vi "Compile Static Commands.vi"(10 "State Loop Data in":T1) -> (2 "State Loop Data out":T1)   [LabVIEW 2023, in "VolatusSeq.lvlib" / "State.lvclass"]
uses:
  State.lvclass
  State.lvclass/State.ctl
  Iteration Actions/Iteration Actions.lvclass
  VolatusSeqConfig/Command Type.ctl
  VolatusSeqConfig/VolatusSeqConfig.lvlib
  Volatus/MessageQ/MessageQ.lvclass
  messages/CmdDigital/Data.ctl
  messages/CmdDigital/CmdDigital.lvlib
  messages/CmdAnalog/Data.ctl
  messages/CmdAnalog/CmdAnalog.lvlib
  Command.ctl
  VolatusSeq.lvlib
  Transition/Transition.lvclass
  Sequence Time.ctl
  State Loop Data.ctl
  Send Type.ctl
  Variables/Variables.lvclass
  lv-vecto/Vecto/Channel DBL/Channel DBL.lvclass
  Format String/Format String.lvclass
  VolatusSeqConfig/Debug Flags.ctl
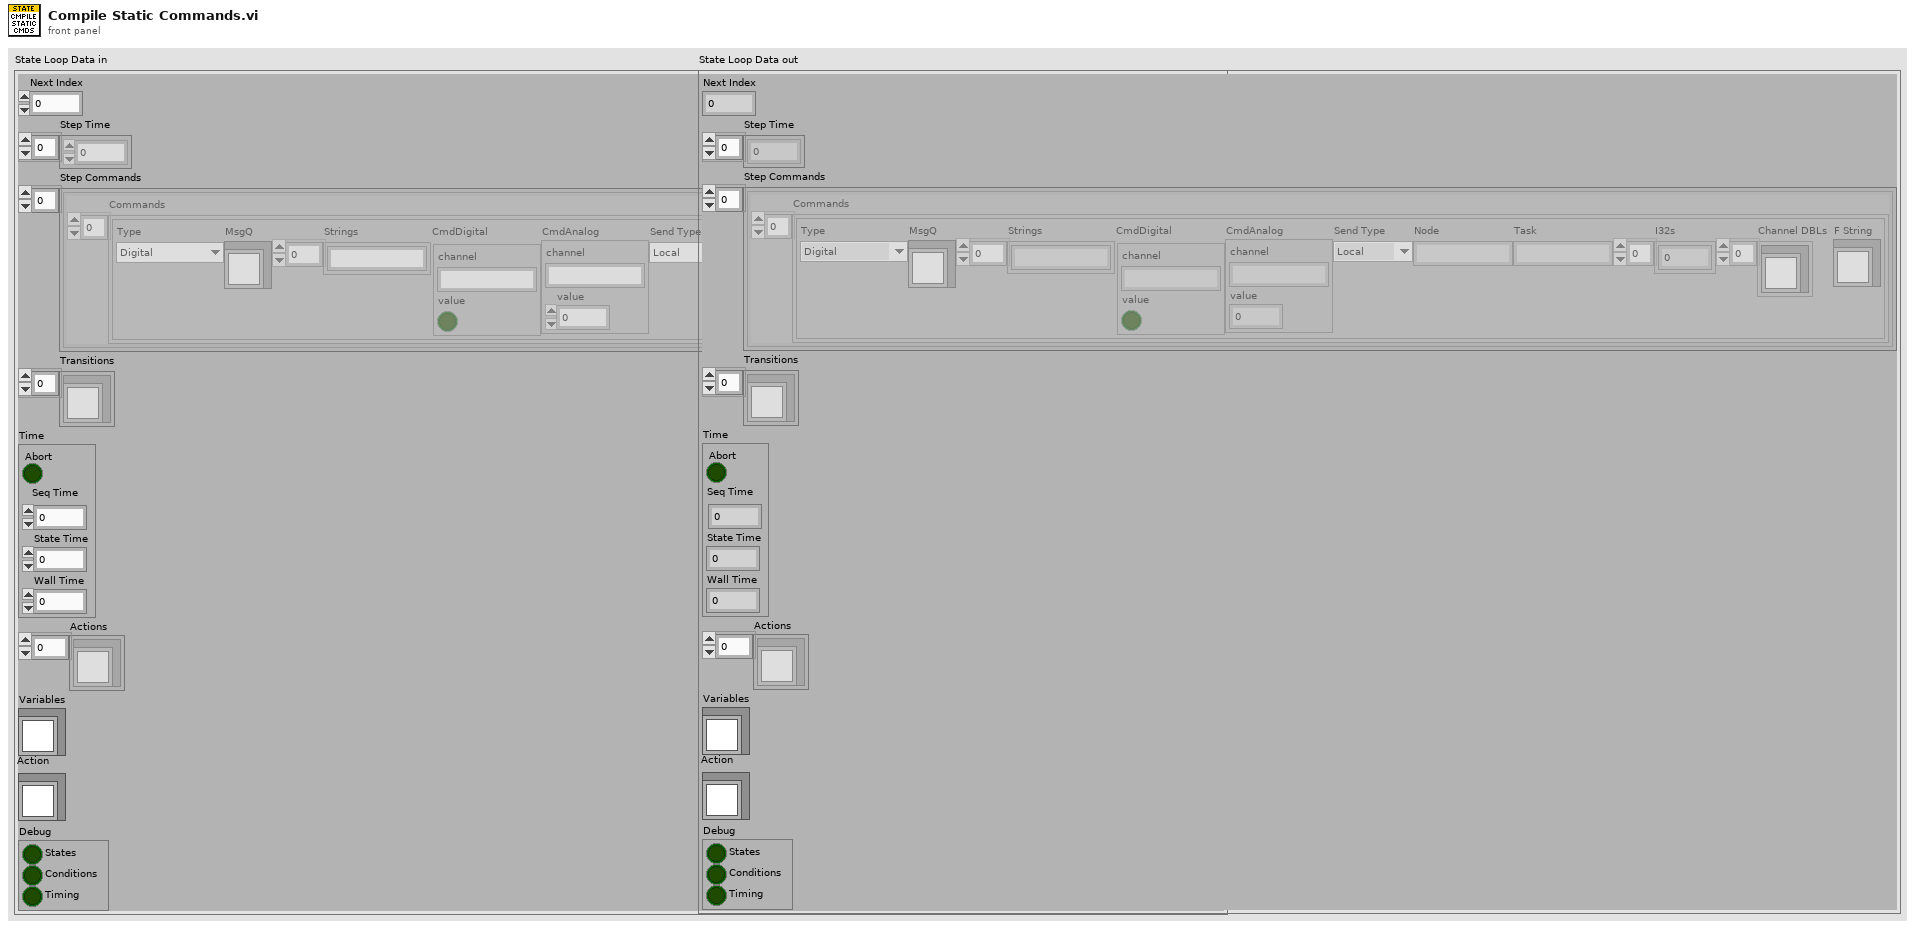
[diagram p1: front panel]
types:
  T1 = typedef "VolatusSeq.lvlib/State.lvclass/State Loop Data.ctl" = cluster{"Next Index":i32, "Step Time":dbl[], "Step Commands":cluster{"Commands":T2[]}[], "Transitions":refnum<class "Transition.lvclass">[], "Time":T7, "Actions":refnum<class "Iteration Actions.lvclass">[], "Variables":refnum<class "Variables.lvclass">, "Action":refnum<class "Iteration Actions.lvclass">, "Debug":T8}
  T2 = typedef "VolatusSeq.lvlib/Command.ctl" = cluster{"Type":T3, "MsgQ":refnum<class "MessageQ.lvclass">, "Strings":string[], "CmdDigital":T4, "CmdAnalog":T5, "Send Type":T6, "Node":string, "Task":string, "I32s":i32[], "Channel DBLs":refnum<class "Channel DBL.lvclass">[], "F String":refnum<class "Format String.lvclass">}
  T3 = typedef "VolatusSeqConfig.lvlib/Command Type.ctl" = enum16{"Digital", "Numeric", "Transition", "Stop", "StartLog", "StopLog", "Start", "Event", "Error", "HTTP", "ResetVar", "IncVar", "DecVar", "SaveVar", "LoadVar", "AddVar", "SubVar", "SetVar", "AddToVar"}
  T4 = typedef "CmdDigital.lvlib/Data.ctl" = cluster{"channel":string, "value":bool}
  T5 = typedef "CmdAnalog.lvlib/Data.ctl" = cluster{"channel":string, "value":dbl}
  T6 = typedef "VolatusSeq.lvlib/Send Type.ctl" = enum16{"Local", "Remote"}
  T7 = typedef "VolatusSeq.lvlib/Sequence Time.ctl" = cluster{"Abort":bool, "Seq Time":dbl, "State Time":dbl, "Wall Time":dbl}
  T8 = typedef "VolatusSeqConfig.lvlib/Debug Flags.ctl" = cluster{"States":bool, "Conditions":bool, "Timing":bool}
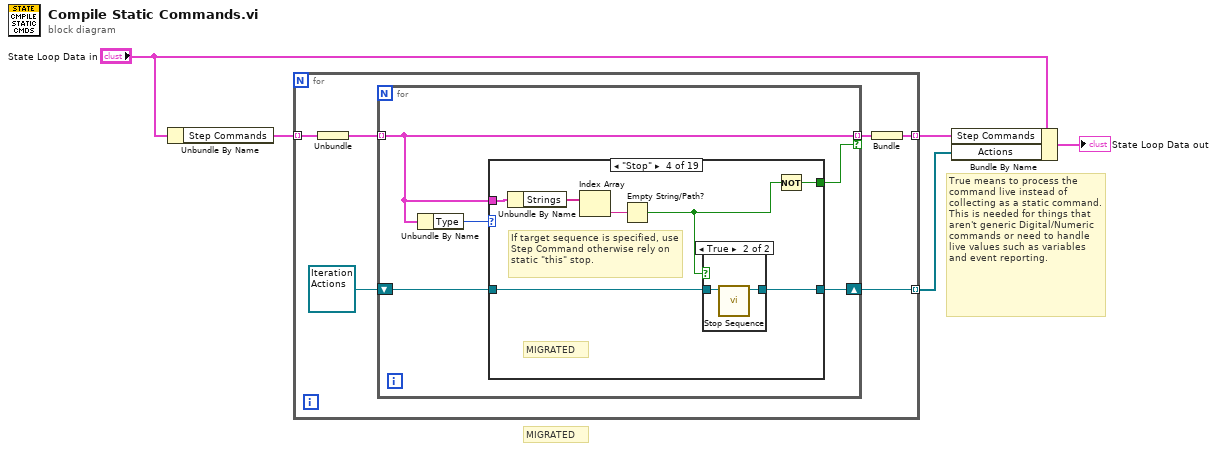
[diagram p0: block diagram]
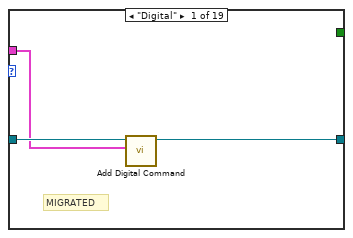
[diagram p2: hidden frame]
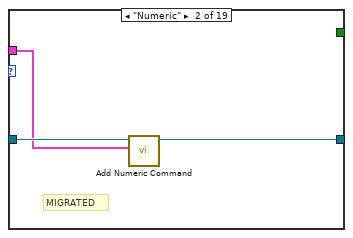
[diagram p3: hidden frame]
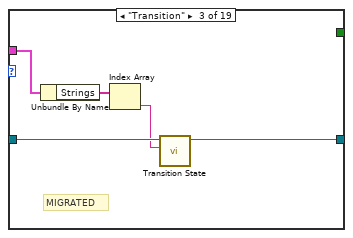
[diagram p4: hidden frame]
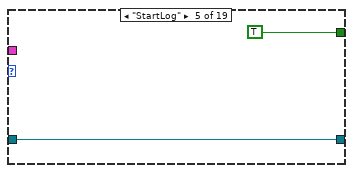
[diagram p6: hidden frame]
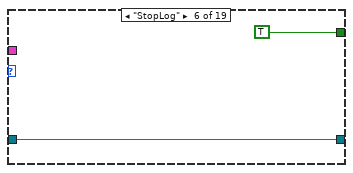
[diagram p7: hidden frame]
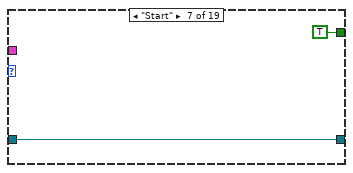
[diagram p8: hidden frame]
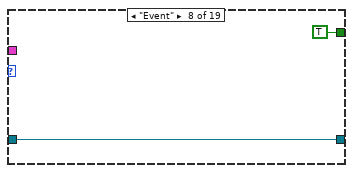
[diagram p9: hidden frame]
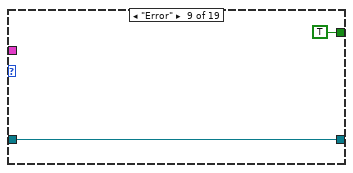
[diagram p10: hidden frame]
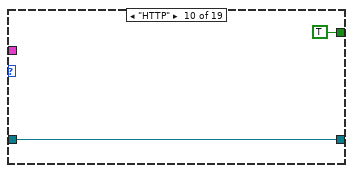
[diagram p11: hidden frame]
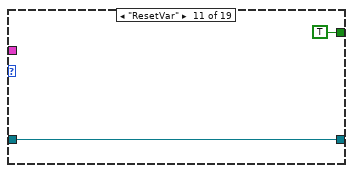
[diagram p12: hidden frame]
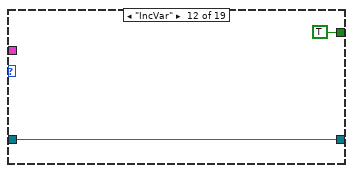
[diagram p13: hidden frame]
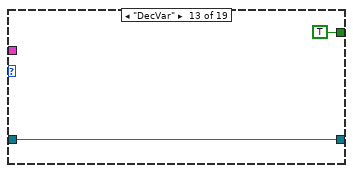
[diagram p14: hidden frame]
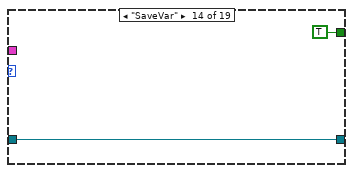
[diagram p15: hidden frame]
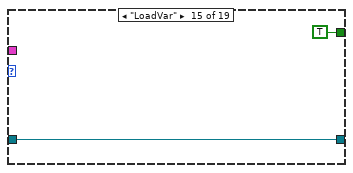
[diagram p16: hidden frame]
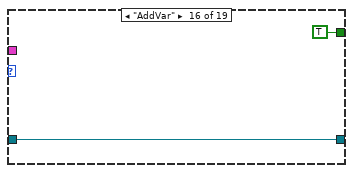
[diagram p17: hidden frame]
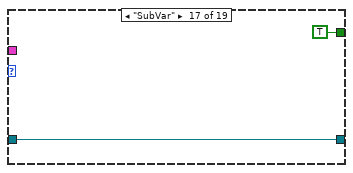
[diagram p18: hidden frame]
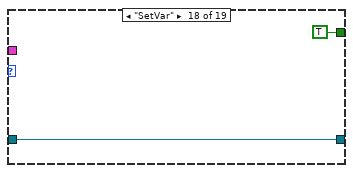
[diagram p19: hidden frame]
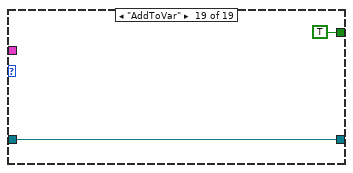
[diagram p20: hidden frame]
diagram:
  # "MIGRATED"
  # "True means to process the command live instead of collecting as a static command. This is needed for things that aren't generic Digital/Numeric commands or need to handle live values such as variables and event reporting."
  n1 = Unbundle By Name("State Loop Data in") -> ("Step Commands"=w3:cluster{"Commands":T2[]}[])
  n2 = for {
    tunnel: w3 -> [w11] mode=indexing
    tunnel: [w7] -> w2 mode=indexing
    tunnel: [w6] -> w1 mode=indexing
    n3 = Unbundle(w11) -> ("Commands"=w10:T2[])
    n4 = for {
      tunnel: w10 -> [w15] mode=indexing
      shift-right: [w13] -> w6
      shift-left: refnum<class "Iteration Actions.lvclass"> refnum ("VolatusSeq.lvlib:Iteration Actions.lvclass") -> [w14]
      tunnel: [w15] -> w8 mode=indexing if=w12
      n5 = Unbundle By Name(w15) -> ("Type"=w16:T3)
      n6 = case shown="\"Stop\"" w16 {
        tunnel: w15 -> [w17 w20 w26 w32 _ _ _ _ _ _ _ _ _ _ _ _ _ _ _]
        tunnel: w14 -> [w19 w22 w27 w34 w39 w41 w43 w45 w47 w49 w51 w53 w55 w57 w59 w61 w63 w65 w67]
        tunnel: [w18 w21 w23 w33 w39 w41 w43 w45 w47 w49 w51 w53 w55 w57 w59 w61 w63 w65 w67] -> w13
        tunnel: [_ _ _ w29 TRUE TRUE TRUE TRUE TRUE TRUE TRUE TRUE TRUE TRUE TRUE TRUE TRUE TRUE TRUE] -> w12
        frame "Digital" {
          # "MIGRATED"
          n7 = call "Add Digital Command.vi"("Command"=w17, "Iteration Actions in"=w19) -> ("Iteration Actions out"=w18:refnum<class "Iteration Actions.lvclass">)  [unwired: 8 in, 1 out]
        }
        frame "Numeric" {
          # "MIGRATED"
          n8 = call "Add Numeric Command.vi"("Command"=w20, "Iteration Actions in"=w22) -> ("Iteration Actions out"=w21:refnum<class "Iteration Actions.lvclass">)  [unwired: 8 in, 1 out]
        }
        frame "Transition" {
          # "MIGRATED"
          n9 = Unbundle By Name(w26) -> ("Strings"=w25:string[])
          n10 = Index Array(array=w25) -> (element=w24:string)  [unwired: 1 in]
          n11 = call "Transition State.vi"("Next State"=w24, "Iteration Actions in"=w27) -> ("Iteration Actions out"=w23:refnum<class "Iteration Actions.lvclass">)  [unwired: 8 in, 1 out]
        }
        frame "Stop" {
          # "MIGRATED"
          # "If target sequence is specified, use Step Command otherwise rely on static \"this\" stop."
          n12 = Unbundle By Name(w32) -> ("Strings"=w31:string[])
          n13 = Index Array(array=w31) -> (element=w30:string)  [unwired: 1 in]
          n14 = Empty String/Path?(string/path=w30) -> (empty?=w28:bool)
          n15 = case shown="True" w28 {
            tunnel: w34 -> [w35 w37]
            tunnel: [w35 w36] -> w33
            frame False {
            }
            frame True {
              n16 = call "Stop Sequence.vi"("Iteration Actions in"=w37) -> ("Iteration Actions out"=w36:refnum<class "Iteration Actions.lvclass">)  [unwired: 9 in, 1 out]
            }
          }
          n17 = Not(x=w28) -> (.not. x?=w29:bool)
        }
        frame "StartLog" {
        }
        frame "StopLog" {
        }
        frame "Start" {
        }
        frame "Event" {
        }
        frame "Error" {
        }
        frame "HTTP" {
        }
        frame "ResetVar" {
        }
        frame "IncVar" {
        }
        frame "DecVar" {
        }
        frame "SaveVar" {
        }
        frame "LoadVar" {
        }
        frame "AddVar" {
        }
        frame "SubVar" {
        }
        frame "SetVar" {
        }
        frame "AddToVar" {
        }
      }
    }
    n18 = Bundle(w8) -> (w7:cluster{T2[]})  [unwired: 1 in]
  }
  n19 = Bundle By Name(cluster="State Loop Data in", "Step Commands"=w2, "Actions"=w1) -> (→"State Loop Data out":T1)
